vi "Add Sensor Asic.vi"(8 "error in (no error)":errorcluster caption="错误输入（无错误）", 10 "asicHandle":i32, 11 "sensorHandle":i32) -> (0 "error out":errorcluster caption="错误输出", 1 "AsicHandle out":i32, 3 "数值":i32)   [LabVIEW 2020]
doc: "extern int __stdcall APSxCreateSensorObject (IN int pgiType, IN char * sensorName, OUT int * sensorHandle); extern int __stdcall APSxAddSensorAsic (int sensorHandle, IN int asicHandle);"
uses:
  APSx.dll/APSx.dll
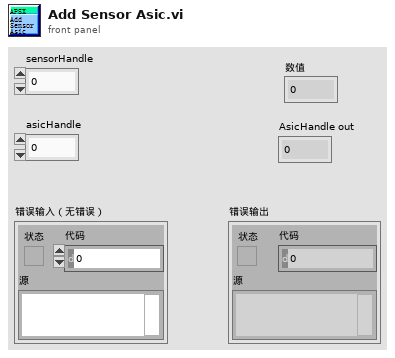
[diagram p1: front panel]
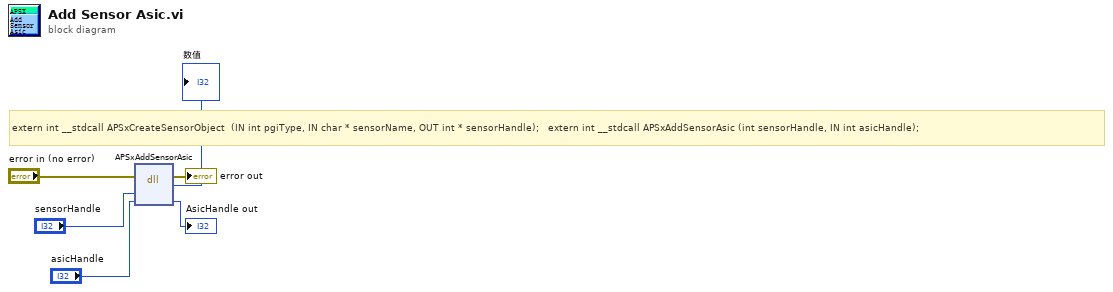
[diagram p0: block diagram]
diagram:
  # "extern int __stdcall APSxCreateSensorObject  (IN int pgiType, IN char * sensorName, OUT int * sensorHandle);   extern int __stdcall APSxAddSensorAsic (int sensorHandle, IN int asicHandle);"
  n1 = dll-call lib="PTH2iabs CUsersFengDesktop传感器对中台传感器对中台labviewSourcesAPSx.dllAPSx.dll" fn="APSxAddSensorAsic"(error in="error in (no error)", "sensorHandle"="sensorHandle", "asicHandle"="asicHandle") -> (error out=→"error out":errorcluster, "返回类型"=→"数值":i32, "asicHandle"=→"AsicHandle out":i32)  [unwired: 3 in, 1 out]
